vi "From Variant.vi"(0 "Obj in":refnum<class "Waveform.lvclass">, 7 "Variant":variant, 9 "Prefix":string, 11 "error in (no error)":errorcluster) -> (4 "Obj out":refnum<class "Waveform.lvclass">, 15 "error out":errorcluster)   [LabVIEW 2020, in "Waveform.lvclass"]
uses:
  Waveform.lvclass
  Waveform.lvclass/Waveform.ctl
  Koop/KObject Class/KObject.lvclass
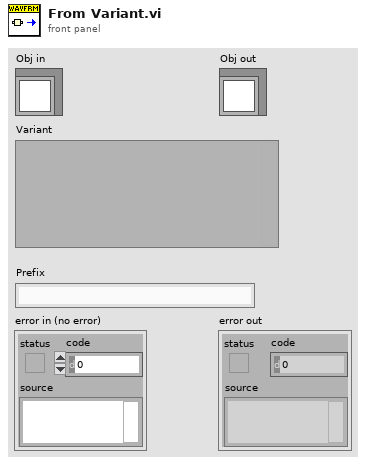
[diagram p1: front panel]
types:
  T1 = typedef "Waveform.lvclass/Serialized.ctl" = cluster{"Numeric":dbl}
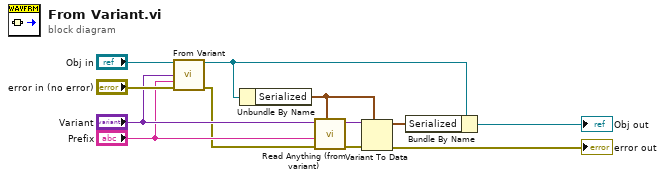
[diagram p0: block diagram]
diagram:
  n1 = call-parent "From Variant.vi"("KObject in"="Obj in", "Variant"="Variant", "Prefix"="Prefix", "error in (no error)"="error in (no error)") -> ("KObject out"=w2:refnum<class "Waveform.lvclass">, "error out"=w3:errorcluster)  [unwired: 10 in]
  n2 = Unbundle By Name(w2) -> ("Serialized"=w5:T1)
  n3 = call "Read Anything (from variant).vi"("Type of Anything"=w5, "Error In"=w3, "Prefix"="Prefix", "Variant Database"="Variant") -> ("Error Out"=w6:errorcluster, "Anything"=w7:variant)  [unwired: 5 in, 1 out]
  n4 = Variant To Data(error in=w6, type=w5, Variant=w7) -> (data=w4:T1, error out=→"error out":errorcluster)
  n5 = Bundle By Name(cluster=w2, "Serialized"=w4) -> (→"Obj out":refnum<class "Waveform.lvclass">)
